vi "ReadDataFromTextFile.vi"(0 "Byte Stream File Refnum":refnum<file>, 1 "number of acquisitions":i32=10) -> (2 "Data Array Read":string[](array[string]), 4 "error out":errorcluster)   [LabVIEW 2012]
doc: "Reads a text file created by the Write to Text File VI in this LLB and plots the data. The VI reads one line at a time, splits off the first (timestamp) column from the subsequent data columns, and converts the data to numbers and plots them. Refer to the sprdsht.llb for an example of the spreadsheet format."
panel:
  in  "error in (no error)":errorcluster
  out "line":i32
  out "data":dbl[](graph)
  out "time":string
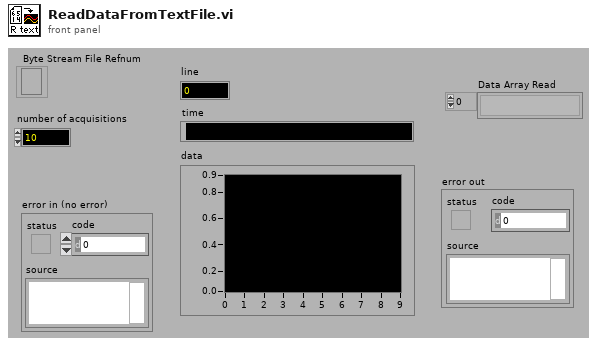
[diagram p1: front panel]
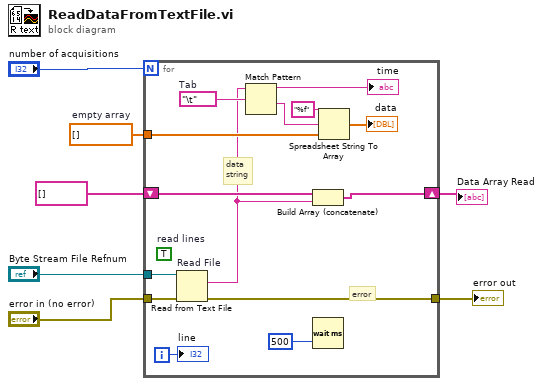
[diagram p0: block diagram]
diagram:
  w7 = dbl[] []  # empty array
  n1 = for {
    N: "number of acquisitions" -> [_]
    tunnel: w7 -> [w12]
    tunnel: "Byte Stream File Refnum" -> [w20]
    tunnel: [w14] -> w3
    tunnel: "error in (no error)" -> [w21]
    shift-right: [w9] -> w1
    shift-left: string[] [] -> [w11]
    i -> [w13]
    w19 = "\t"  # Tab
    (unwired) TRUE  # read lines
    # "data \nstring"
    # "error"
    n2 = Read from Text File "Read File"(file (use dialog)=w20, error in=w21) -> (text=w10:string, error out=w14:errorcluster)  [unwired: 4 out]
    n3 = Match Pattern(string=w10, regular expression=w19) -> (before substring=→"time":string, after substring=w17:string)  [unwired: 3 out]
    n4 = Build Array (concatenate)(w11, w10) -> (w9:string[])
    n5 = Wait (ms)(milliseconds to wait=u32 500) -> ()  [unwired: 1 out]
    n6 = Spreadsheet String To Array(format string="%f", spreadsheet string=w17, array type (2D Dbl)=w12) -> (array=→"data":dbl[])  [unwired: 1 out]
    "line" <- w13
  }
  "error out" <- w3
  "Data Array Read" <- w1
